vi "Elu.vi"(1 "alpha":dbl=1.0 min=1.0 step=0.01 format="%#_13g", 3 "Z":dbl) -> (0 "Elu(Z)":dbl)   [LabVIEW 2020]
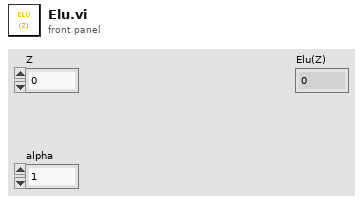
[diagram p1: front panel]
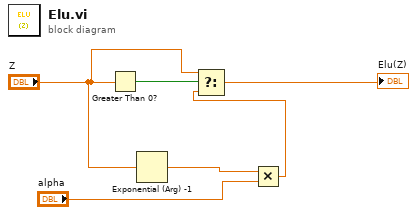
[diagram p0: block diagram]
diagram:
  n1 = Greater Than 0?(x="Z") -> (x > 0?=w6:bool)
  n2 = Exponential (Arg) -1(1:"Z") -> (0:w4:dbl)
  n3 = Multiply(x=w4, y="alpha") -> (x*y=w2:dbl)
  n4 = Select(t="Z", s=w6, f=w2) -> (s? t:f=→"Elu(Z)":dbl)
